vi "Timestamp.vi"() -> (3 "Timestamp":string)   [LabVIEW 2022 SP3]
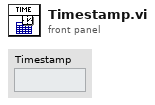
[diagram p1: front panel]
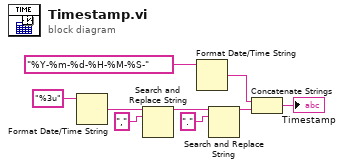
[diagram p0: block diagram]
diagram:
  n1 = Format Date/Time String(time format string (%c)="%3u") -> (date/time string=w9:string)  [unwired: 2 in]
  n2 = Search and Replace String(input string=w9, search string=",") -> (result string=w2:string)  [unwired: 6 in, 3 out]
  n3 = Format Date/Time String(time format string (%c)="%Y-%m-%d-%H-%M-%S-") -> (date/time string=w8:string)  [unwired: 2 in]
  n4 = Search and Replace String(input string=w2, search string=".") -> (result string=w1:string)  [unwired: 6 in, 3 out]
  n5 = Concatenate Strings(w8, w1) -> (→"Timestamp":string)
